vi "WriteReadWait.vi"(5 "Read Value":bool=TRUE, 6 "Numeric":dbl, 7 "Write Value":bool=TRUE, 8 "error in (no error)":errorcluster, 9 "Read":i32, 10 "Write":i32, 11 "I-O in":refnum<class "I-O.lvclass">) -> (0 "error out":errorcluster, 3 "I-O out":refnum<class "I-O.lvclass">)   [LabVIEW 2021, in "I-O.lvclass"]
uses:
  I-O.lvclass
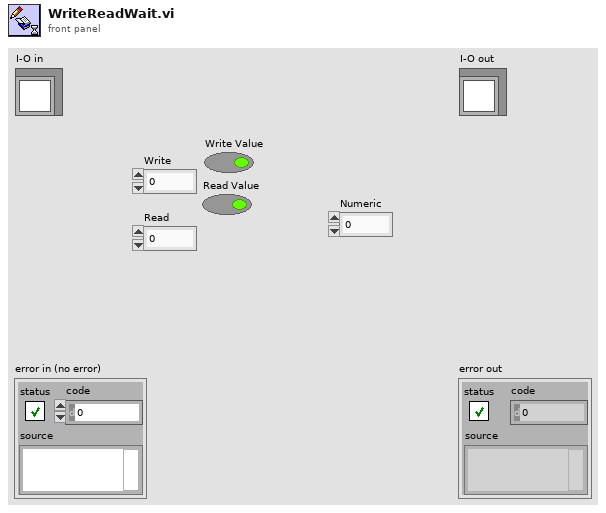
[diagram p1: front panel]
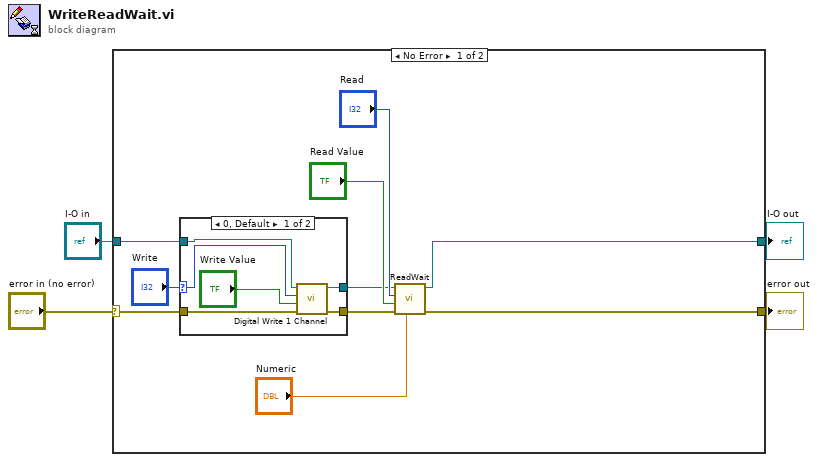
[diagram p0: block diagram]
diagram:
  n1 = case shown="No Error" "error in (no error)" {
    selector: "error in (no error)" -> [w11 w24]
    tunnel: [w12 w24] -> w3
    tunnel: [w13 w23] -> w1
    tunnel: "I-O in" -> [w14 w23]
    frame No Error {
      n2 = case shown="0, Default" "Write" {
        selector: "Write" -> [w15 _]
        tunnel: w14 -> [w20 w21]
        tunnel: w11 -> [w19 w22]
        tunnel: [w17 w21] -> w8
        tunnel: [w16 w22] -> w7
        frame 0, Default {
          n3 = call-dynamic "Digital Write 1 Channel.vi"("error constant"=w19, "Value"="Write Value", "Channel"=w15, "I-O.lvclass"=w20) -> ("error IO"=w16:errorcluster, "I-O.lvclass 2"=w17:refnum<class "I-O.lvclass">)  [unwired: 6 in]
        }
        frame -1 {
        }
      }
      n4 = call "ReadWait.vi"("Numeric"="Numeric", "error in (no error)"=w7, "Value"="Read Value", "Read"="Read", "I-O in"=w8) -> ("error out"=w12:errorcluster, "I-O out"=w13:refnum<class "I-O.lvclass">)  [unwired: 5 in]
    }
    frame Error {
    }
  }
  "error out" <- w3
  "I-O out" <- w1
